vi "wave crest factor analyzer-Get VI path.vi"(8 "File name":string) -> (0 "appended path":path, 1 "Is exe?":bool, 2 "Current VI Folder":path)   [LabVIEW 2014]
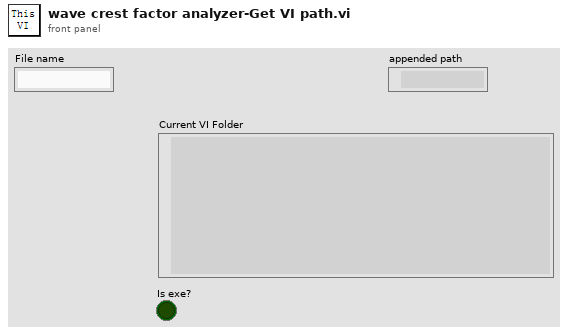
[diagram p1: front panel]
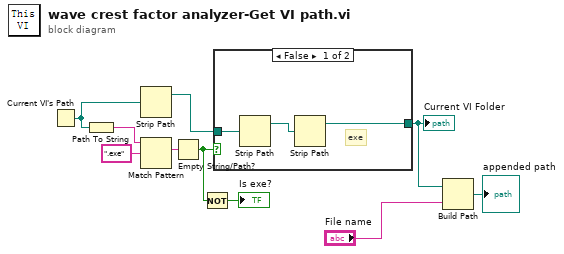
[diagram p0: block diagram]
diagram:
  n1 = Current VI's Path() -> (path=w7:path)
  n2 = Path To String(path=w7) -> (string=w10:string)
  n3 = Strip Path(path=w7) -> (stripped path=w6:path)  [unwired: 1 out]
  n4 = Match Pattern(string=w10, regular expression=".exe") -> (match substring=w8:string)  [unwired: 1 in, 3 out]
  n5 = Empty String/Path?(string/path=w8) -> (empty?=w4:bool)
  n6 = Not(x=w4) -> (.not. x?=→"Is exe?":bool)
  n7 = case shown="False" w4 {
    tunnel: w6 -> [w13 w14]
    tunnel: [w11 w14] -> w3
    frame False {
      # "exe"
      n8 = Strip Path(path=w13) -> (stripped path=w12:path)  [unwired: 1 out]
      n9 = Strip Path(path=w12) -> (stripped path=w11:path)  [unwired: 1 out]
    }
    frame True {
      # "vi"
    }
  }
  "Current VI Folder" <- w3
  n10 = Build Path(base path=w3, name or relative path="File name") -> (appended path=→"appended path":path)
